vi "seriesName.get.vi"(8 "error in (no error)":errorcluster, 11 "timestampMetadata in":refnum<class "timestampMetadata.lvclass">) -> (0 "error out":errorcluster, 2 "seriesName":string, 3 "timestampMetadata out":refnum<class "timestampMetadata.lvclass">)   [LabVIEW 2020, in "timestampMetadata.lvclass"]
uses:
  timestampMetadata.lvclass
  timestampMetadata.lvclass/timestampMetadata.ctl
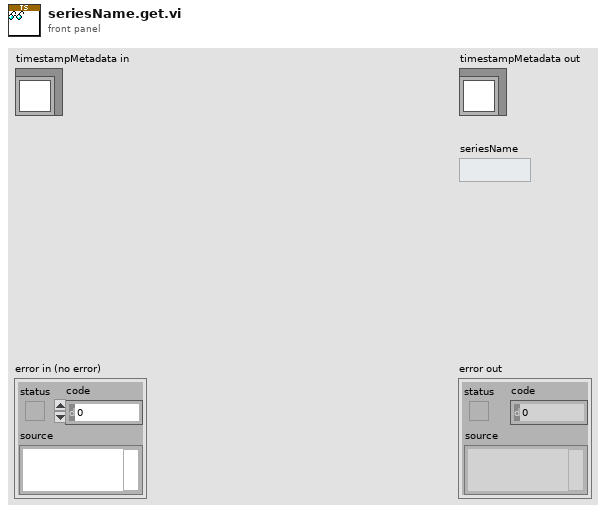
[diagram p1: front panel]
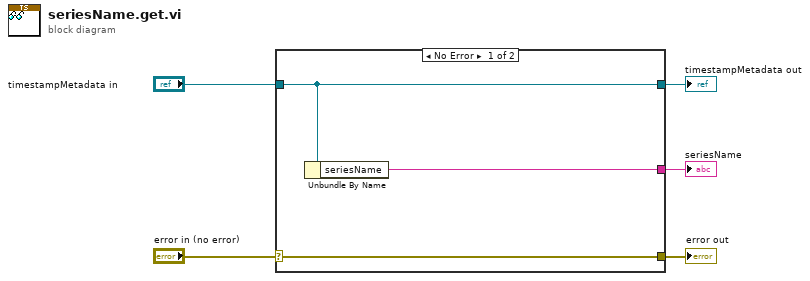
[diagram p0: block diagram]
diagram:
  n1 = case shown="No Error" "error in (no error)" {
    selector: "error in (no error)" -> [w8 w9]
    tunnel: [w8 w9] -> w4
    tunnel: [w7 w10] -> w2
    tunnel: "timestampMetadata in" -> [w7 w10]
    tunnel: [w6 _] -> w1
    frame No Error {
      n2 = Unbundle By Name(w7) -> ("seriesName"=w6:string)
    }
    frame Error {
    }
  }
  "error out" <- w4
  "timestampMetadata out" <- w2
  "seriesName" <- w1
